vi "update.vi"(8 "error in (no error)":errorcluster, 11 "DomeController in":refnum<class "DomeController.lvclass">) -> (0 "error out":errorcluster, 1 "relative seconds":dbl format="%_19f", 2 "shortStatus out":T1 {"azimuthAngle" min=0.0 max=360.0; "dropoutDoorOpeningPercentage" min=0.0 max=100.0; "mainDoorOpeningPercentage" min=0.0 max=100.0}, 3 "DomeController out":refnum<class "DomeController.lvclass">)   [LabVIEW 2016, in "DomeController.lvclass"]
uses:
  DomeController.lvclass
  domeCommunicator/ComTypedefs/shortStatus.ctl
  domeCommunicator/ComTypedefs/openingStates.ctl
  IDome/domeTypedefs/openingPercentage.ctl
  domeCommunicator/ComTypedefs/sensorCode.ctl
  domeCommunicator/ComTypedefs/azimimuthPositionStatus.ctl
  IDome/domeTypedefs/azimuth.ctl
  IDome/domeTypedefs/direction.ctl
  IDome/domeTypedefs/domeState.ctl
  IDome/domeTypedefs/motionDirection.ctl
  IDome/domeTypedefs/openingMotion.ctl
  DomeController.lvclass/DomeController.ctl
  domeCommunicator/ATDomeCommunicator.lvclass
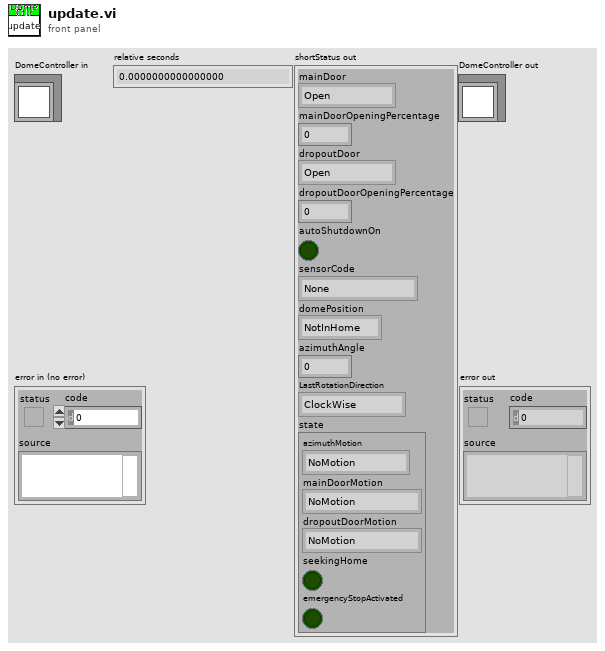
[diagram p1: front panel]
types:
  T1 = typedef "shortStatus.ctl" = cluster{"mainDoor":T2, "mainDoorOpeningPercentage":T3, "dropoutDoor":T2, "dropoutDoorOpeningPercentage":T3, "autoShutdownOn":bool, "sensorCode":T4, "domePosition":T5, "azimuthAngle":T6, "LastRotationDirection":T7, "state":T8}
  T2 = typedef "openingStates.ctl" = enum16{"Open", "Shut", "Ajar"}
  T3 = typedef "openingPercentage.ctl" = dbl
  T4 = typedef "sensorCode.ctl" = enum16{"None", "RainSnowSensorTriggered", "CloudSensorTriggered", "BothSensorsTriggered"}
  T5 = typedef "azimimuthPositionStatus.ctl" = enum16{"NotInHome", "Home"}
  T6 = typedef "azimuth.ctl" = dbl
  T7 = typedef "direction.ctl" = enum16{"ClockWise", "CounterClockWise"}
  T8 = typedef "domeState.ctl" = cluster{"azimuthMotion":T9, "mainDoorMotion":T10, "dropoutDoorMotion ":T10, "seekingHome":bool, "emergencyStopActivated":bool}
  T9 = typedef "motionDirection.ctl" = enum16{"NoMotion", "MovingClockWise", "MovingCounterClockWise"}
  T10 = typedef "openingMotion.ctl" = enum16{"NoMotion", "Opening", "Closing"}
  T11 = typedef "deviceStatus.ctl" = cluster{"status":T12, "statusMessage":string}
  T12 = typedef "statusEnum.ctl" = enum16{"OK", "TIMEOUT", "MSGERROR"}
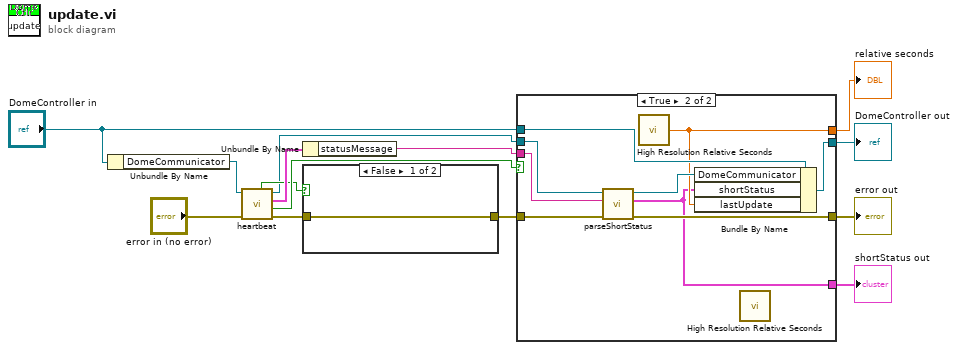
[diagram p0: block diagram]
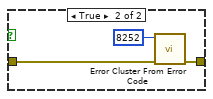
[diagram p2: hidden frame]
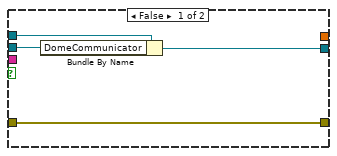
[diagram p3: hidden frame]
diagram:
  n1 = Unbundle By Name("DomeController in") -> ("DomeCommunicator"=w14:refnum<class "ATDomeCommunicator.lvclass">)
  n2 = call-dynamic "heartbeat.vi"("error in (no error)"="error in (no error)", "tcpDevice in"=w14) -> ("error out"=w8:errorcluster, "newValue"=w10:bool, "status"=w9:T11, "tcpDevice out"=w6:refnum<class "ATDomeCommunicator.lvclass">, "timeout?"=w7:bool)  [unwired: 5 in]
  n3 = Unbundle By Name(w9) -> ("statusMessage"=w5:string)
  n4 = case shown="False" w7 {
    tunnel: w8 -> [w15 w18]
    tunnel: [w15 w17] -> w4
    frame False {
    }
    frame True {
      n5 = call <vilib>:"Error Cluster From Error Code.vi"("error in (no error)"=w18, "error code (0)"=8252) -> ("error out"=w17:errorcluster)  [unwired: 7 in]
    }
  }
  n6 = case shown="True" w10 {
    tunnel: "DomeController in" -> [w20 w31]
    tunnel: [w19 w30] -> w11
    tunnel: w6 -> [w21 w29]
    tunnel: w5 -> [_ w28]
    tunnel: w4 -> [w22 w27]
    tunnel: [w22 w26] -> w3
    tunnel: [_ w24] -> w2
    tunnel: [_ w23] -> w1
    frame False {
      n7 = Bundle By Name(cluster=w20, "DomeCommunicator"=w21) -> (w19:refnum<class "DomeController.lvclass">)
    }
    frame True {
      n8 = call "parseShortStatus.vi"("error in (no error)"=w27, "shortStatusString"=w28, "DomeCommunicator in"=w29) -> ("error out"=w26:errorcluster, "shortStatus out"=w23:T1, "DomeCommunicator out"=w25:refnum<class "ATDomeCommunicator.lvclass">)  [unwired: 6 in]
      n9 = call <vilib>:"High Resolution Relative Seconds.vi"() -> ("relative seconds"=w24:dbl)
      n10 = Bundle By Name(cluster=w31, "DomeCommunicator"=w25, "shortStatus"=w23, "lastUpdate"=w24) -> (w30:refnum<class "DomeController.lvclass">)
      n11 = call <vilib>:"High Resolution Relative Seconds.vi"() -> ()  [unwired: 1 out]
    }
  }
  "error out" <- w3
  "DomeController out" <- w11
  "shortStatus out" <- w1
  "relative seconds" <- w2
